vi "Send Stop Event.vi"(8 "error in (no error)":errorcluster, 11 "Generic Instrument.lvlib:Generic Instrument.lvclass":refnum<class "Generic Instrument.lvclass">) -> (0 "error out":errorcluster, 3 "Generic Instrument out":refnum<class "Generic Instrument.lvclass">)   [LabVIEW 2014, in "Generic Instrument.lvlib" / "Generic Instrument.lvclass"]
uses:
  Generic Instrument.lvclass
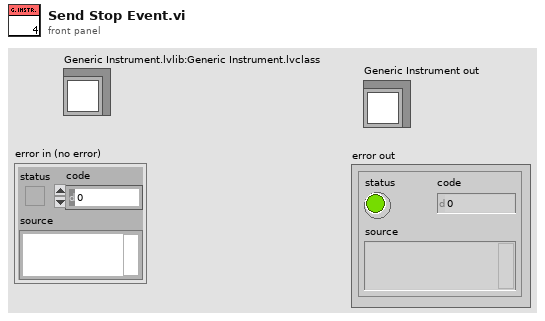
[diagram p1: front panel]
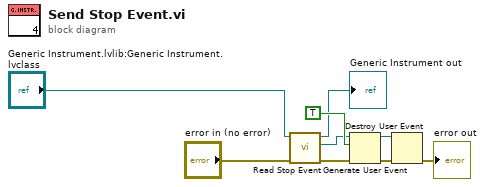
[diagram p0: block diagram]
diagram:
  n1 = call-dynamic "Read Stop Event.vi"("error in (no error)"="error in (no error)", "Generic Instrument in"="Generic Instrument.lvlib:Generic Instrument.lvclass") -> ("error out"=w4:errorcluster, "Stop Event"=w5:refnum<user-event>, "Generic Instrument out"=→"Generic Instrument out":refnum<class "Generic Instrument.lvclass">)  [unwired: 7 in]
  n2 = Generate User Event(user event=w5, event data cluster=TRUE ("event data"), error in=w4) -> (user event out=w7:refnum<user-event>, error out=w6:errorcluster)  [unwired: 1 in]
  n3 = Destroy User Event(user event=w7, error in=w6) -> (error out=→"error out":errorcluster)
